vi "Shoot.vi"(5 "Auto_Enable":bool, 6 "Aimed?":bool, 8 "Stopped?":bool, 9 "Yaw":dbl, 11 "Auto_Selection":T1=enum."Ramparts") -> (0 "Far_Shoot":bool, 1 "Hunt":bool, 2 "Shoot":bool, 3 "Auto_Aim":bool, 4 "Lower_Arm":bool, 7 "Auto_Aim_Enable":bool, 10 "Stage":bool)   [LabVIEW 2015]
uses:
  Auto_Selection.ctl
  Shoot_Type_Def.ctl
panel:
  out "error":errorcluster={"status"=TRUE, "code"=0, "source"="DID NOT DRIVE THE DISTANCE : ROUGH TERRAIN"}
  in  "Clear Error":bool
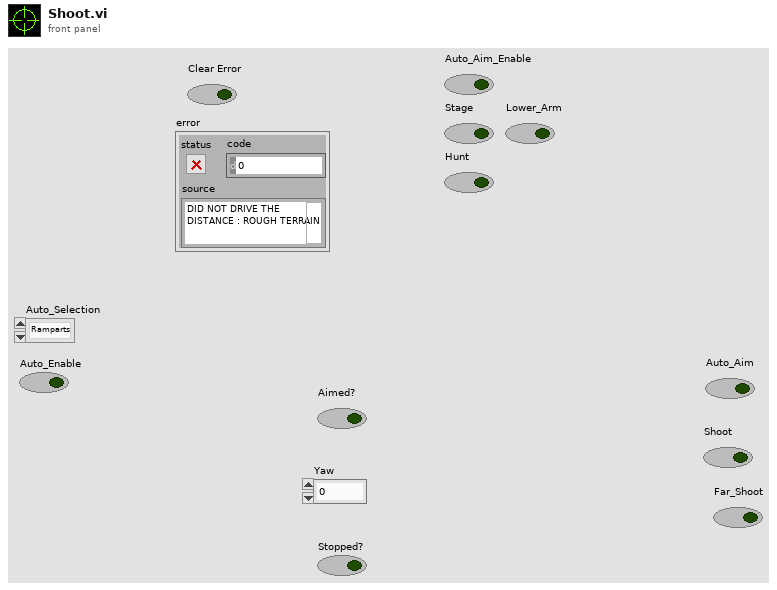
[diagram p1: front panel]
types:
  T1 = typedef "Auto_Selection.ctl" = enum16{"Low Bar", "Rough Terrain", "Rock Wall", "Ramparts", "Moat", "Cheval de Frise", "Portcullis", "None", "One  Ball", "Shoot"}
  T2 = typedef "Shoot_Type_Def.ctl" = enum16{"Off", "Stop", "Shoot", "Aim", "Aim_2", "Delay", "Delay_1"}
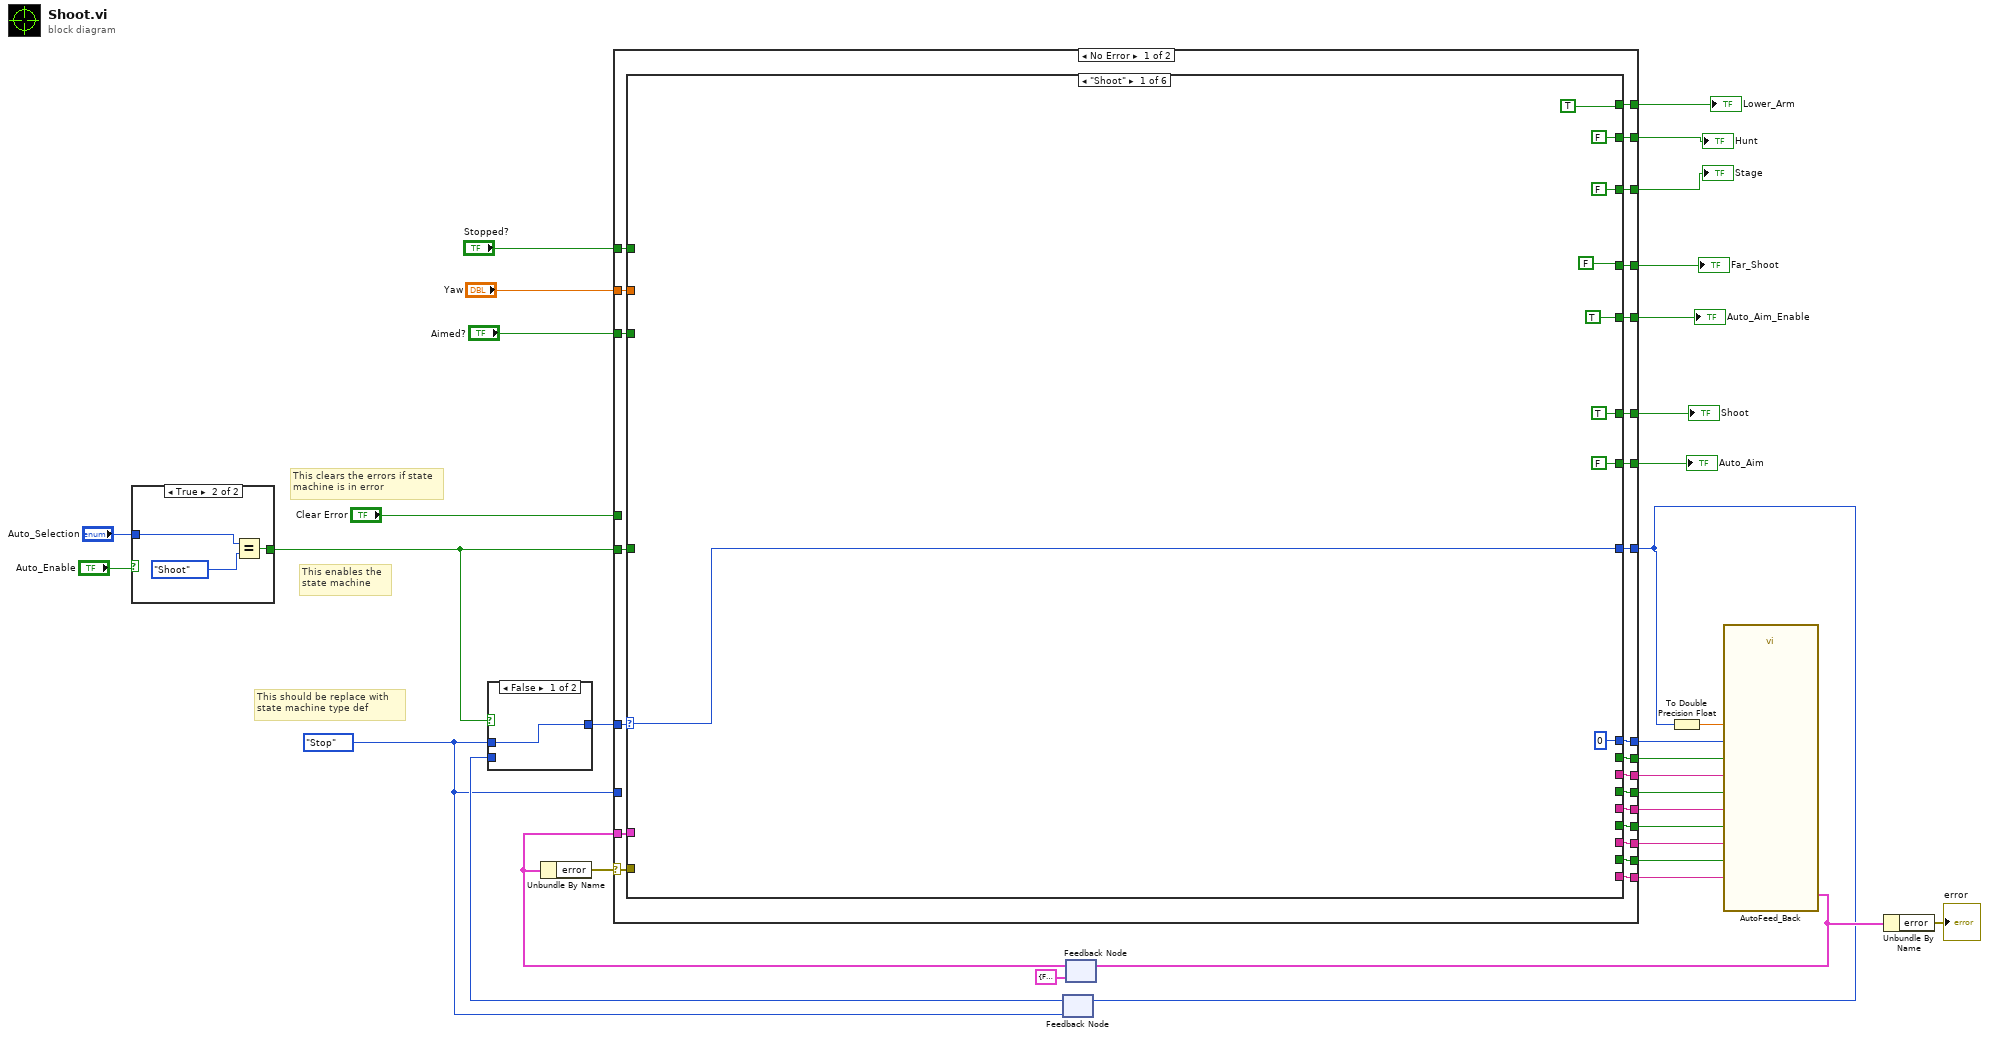
[diagram p0: block diagram]
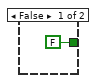
[diagram p2: hidden frame]
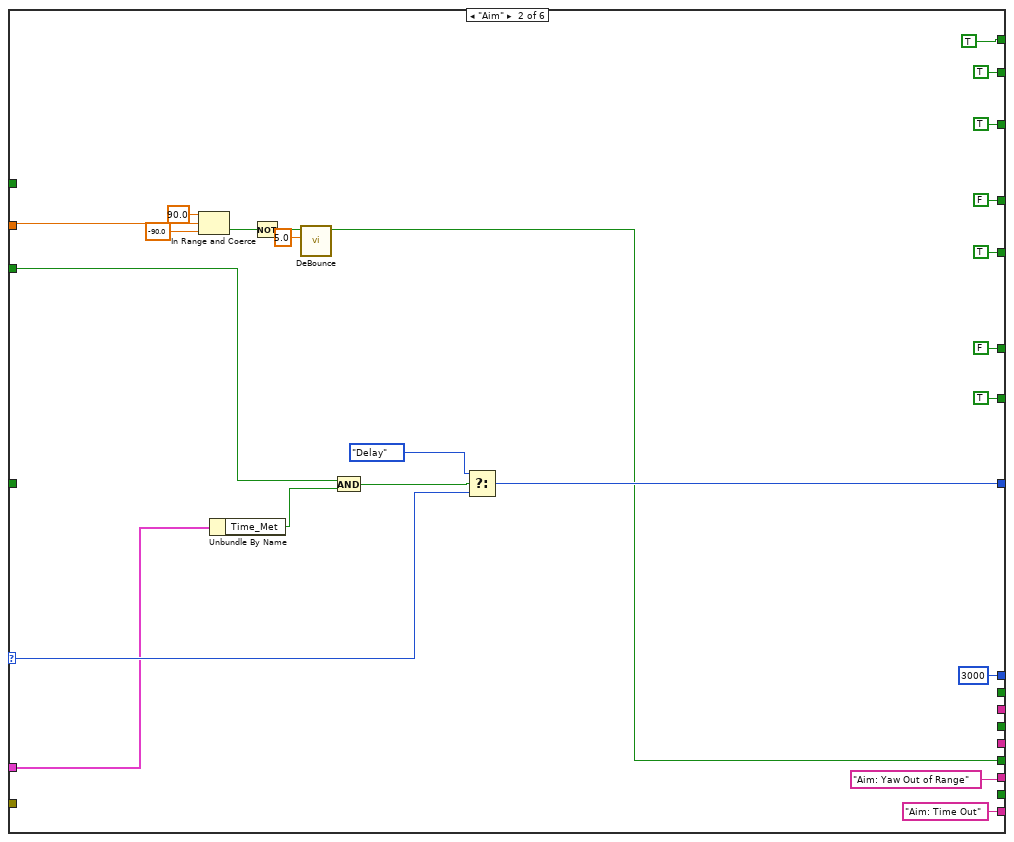
[diagram p4: hidden frame]
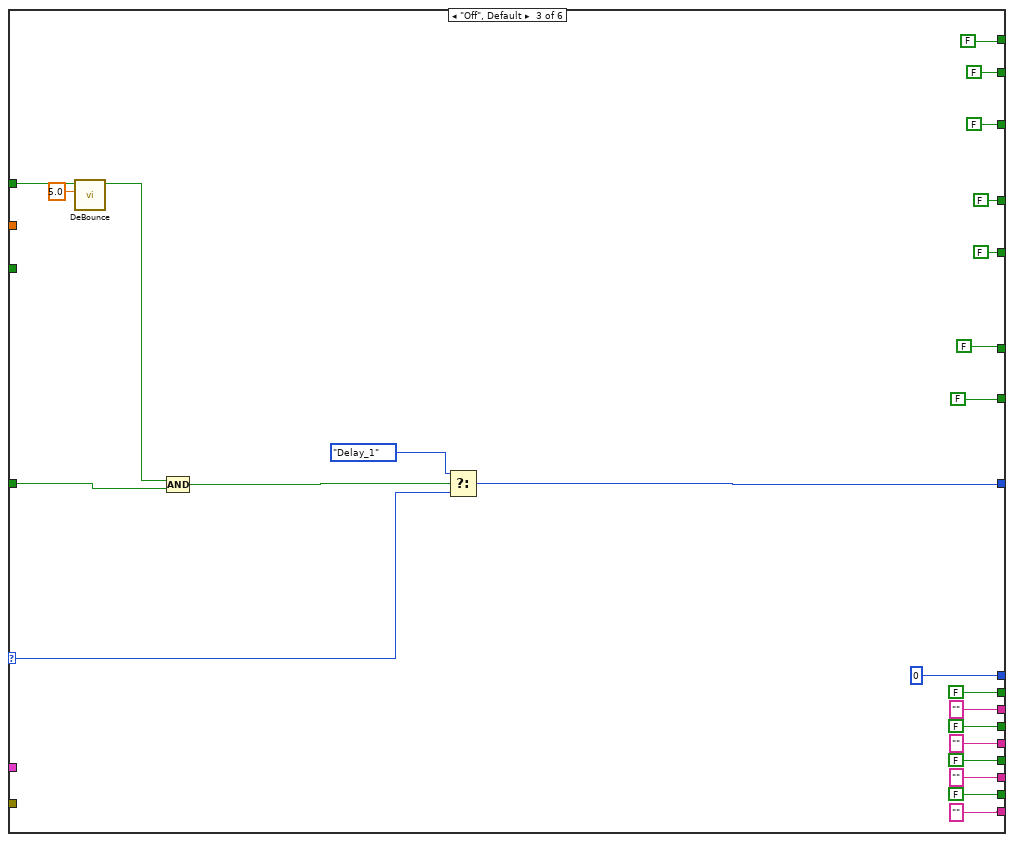
[diagram p5: hidden frame]
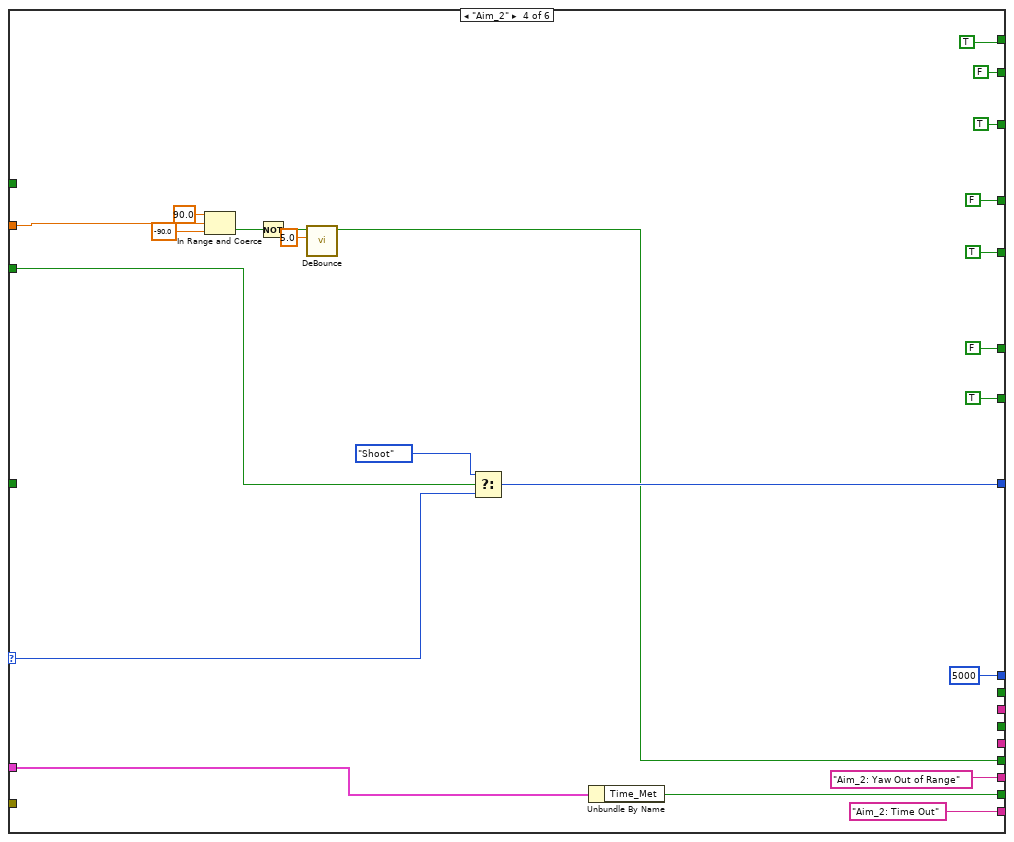
[diagram p6: hidden frame]
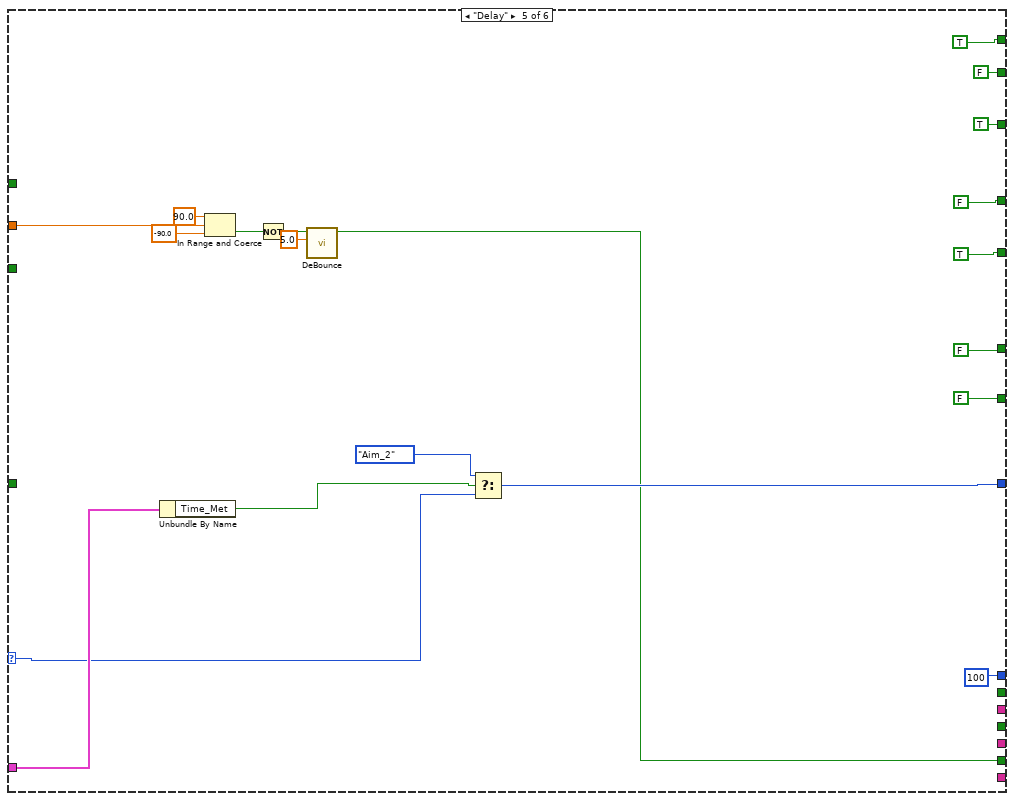
[diagram p7: hidden frame]
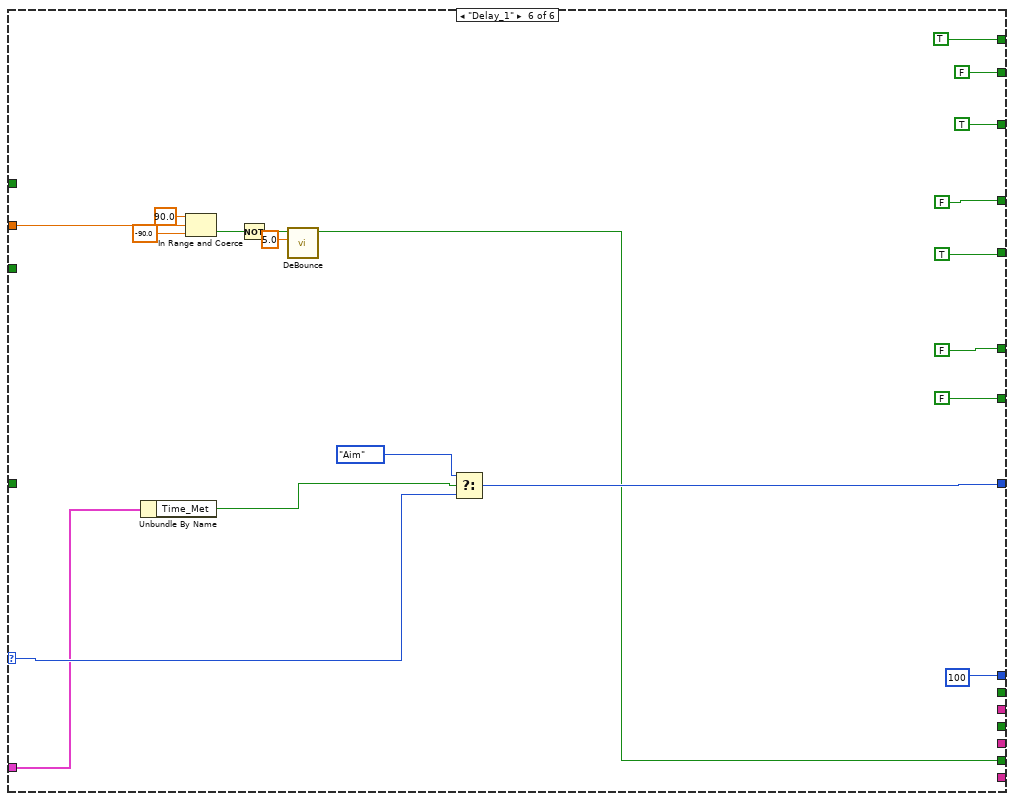
[diagram p8: hidden frame]
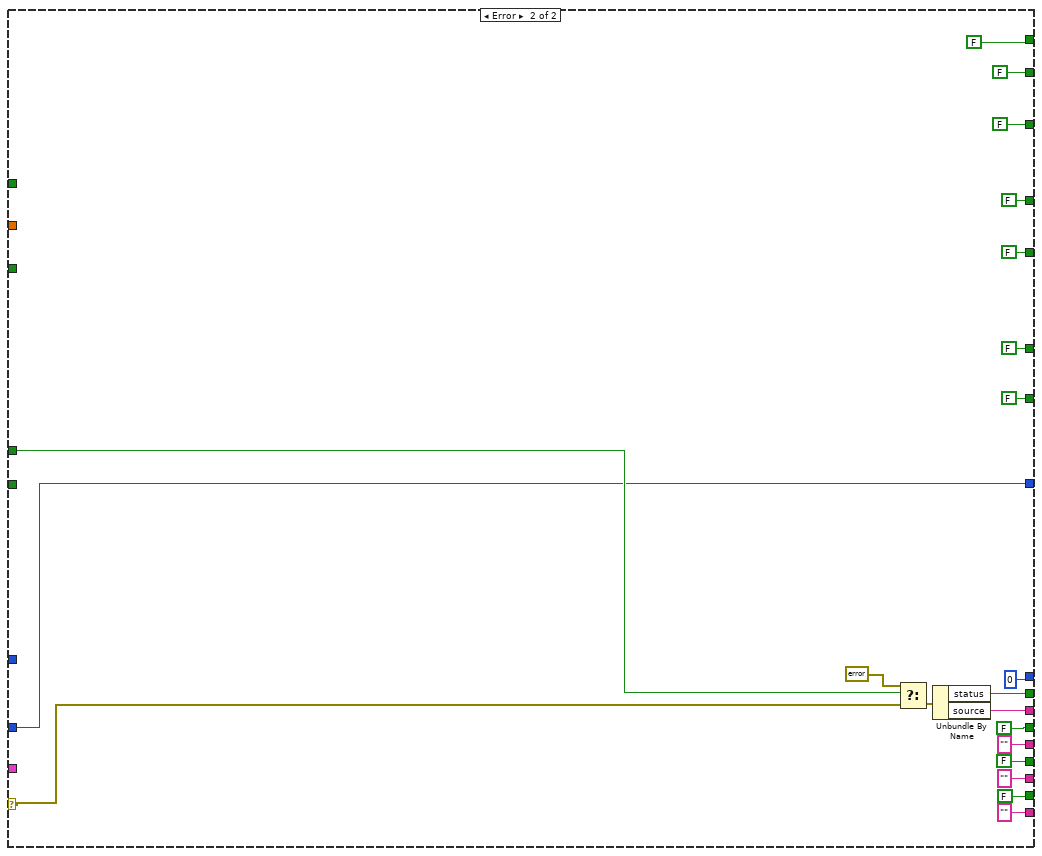
[diagram p9: hidden frame]
diagram:
  w8 = Shoot_Type_Def."Stop"
  # "This clears the errors if state \nmachine is in error"
  # "This enables the \nstate machine"
  # "This should be replace with \nstate machine type def"
  n1 = case shown="True" "Auto_Enable" {
    tunnel: "Auto_Selection" -> [_ w36]
    tunnel: [FALSE w37] -> w25
    frame False {
    }
    frame True {
      n2 = Equal?(x=w36, y=Auto_Selection."Shoot" ("Auto_Selection")) -> (x = y?=w37:bool)
    }
  }
  n3 = feedback #1(w8) -> (w27:T2)
  n4 = case shown="False" w25 {
    tunnel: w8 -> [w38 _]
    tunnel: [w38 w39] -> w28
    tunnel: w27 -> [_ w39]
    frame False {
    }
    frame True {
    }
  }
  n5 = feedback #2(cluster{"Time_Met":bool, "error ":errorcluster} {"Time_Met"=FALSE, "error "={"status"=FALSE, "code"=0, "source"=""}} ("Feedback_State")) -> (w29:cluster{"Time_Met":bool, "error ":errorcluster})
  n6 = Unbundle By Name(w29) -> ("error"=w31:errorcluster)
  n7 = case shown="No Error" w31 {
    selector: w31 -> [w60 w203]
    tunnel: [w63 w200] -> w12
    tunnel: [w62 0] -> w33
    tunnel: "Clear Error" -> [_ w202]
    tunnel: w29 -> [w61 _]
    tunnel: w25 -> [w59 _]
    tunnel: w28 -> [w58 _]
    tunnel: w8 -> [_ w200]
    tunnel: [w57 w198] -> w22
    tunnel: [w56 FALSE] -> w21
    tunnel: [w55 FALSE] -> w20
    tunnel: [w54 FALSE] -> w19
    tunnel: [w53 w197] -> w18
    tunnel: [w52 ""] -> w17
    tunnel: [w51 ""] -> w16
    tunnel: [w50 ""] -> w15
    tunnel: [w49 FALSE] -> w11
    tunnel: [w48 FALSE] -> w10
    tunnel: "Aimed?" -> [w47 _]
    tunnel: "Yaw" -> [w46 _]
    tunnel: [w45 FALSE] -> w6
    tunnel: "Stopped?" -> [w44 _]
    tunnel: [w43 FALSE] -> w4
    tunnel: [w42 FALSE] -> w3
    tunnel: [w41 FALSE] -> w2
    tunnel: [w40 FALSE] -> w1
    frame No Error {
      n8 = case shown="\"Shoot\"" w58 {
        selector: w58 -> [w68 w93 w119 w135 w149 w166]
        tunnel: [0 3000 0 5000 100 100] -> w62
        tunnel: [w68 w92 w118 w133 w153 w169] -> w63
        tunnel: w61 -> [_ w90 _ w134 w150 w165]
        tunnel: w60 -> [_ _ _ _ _ _]
        tunnel: w59 -> [_ _ w105 _ _ _]
        tunnel: [_ _ FALSE _ _ _] -> w57
        tunnel: [_ _ FALSE _ _ _] -> w56
        tunnel: [_ w82 FALSE w126 w152 w168] -> w55
        tunnel: [_ _ FALSE w124 _ _] -> w54
        tunnel: [_ _ "" _ _ _] -> w53
        tunnel: [_ _ "" _ _ _] -> w52
        tunnel: [_ "Aim: Yaw Out of Range" "" "Aim_2: Yaw Out of Range" _ _] -> w51
        tunnel: [_ "Aim: Time Out" "" "Aim_2: Time Out" _ _] -> w50
        tunnel: [FALSE TRUE FALSE TRUE FALSE FALSE] -> w49
        tunnel: [TRUE FALSE FALSE FALSE FALSE FALSE] -> w48
        tunnel: w47 -> [_ w76 _ w136 _ _]
        tunnel: w46 -> [_ w88 _ w137 w148 w164]
        tunnel: [TRUE TRUE FALSE TRUE TRUE TRUE] -> w45
        tunnel: w44 -> [_ _ w103 _ _ _]
        tunnel: [FALSE FALSE FALSE FALSE FALSE FALSE] -> w43
        tunnel: [FALSE TRUE FALSE FALSE FALSE FALSE] -> w42
        tunnel: [FALSE TRUE FALSE TRUE TRUE TRUE] -> w41
        tunnel: [TRUE TRUE FALSE TRUE TRUE TRUE] -> w40
        frame "Shoot" {
        }
        frame "Aim" {
          n9 = In Range and Coerce(upper limit=90.0, x=w88, lower limit=-90.0) -> (In Range?=w85:bool)  [unwired: 1 out]
          n10 = Unbundle By Name(w90) -> ("Time_Met"=w77:bool)
          n11 = Not(x=w85) -> (.not. x?=w84:bool)
          n12 = call "DeBounce.vi"("DB_Count"=5.0, "Value"=w84) -> ("BD_Value"=w82:bool)  [unwired: 9 in]
          n13 = And(x=w76, y=w77) -> (x .and. y?=w78:bool)
          n14 = Select(t=Shoot_Type_Def."Delay", s=w78, f=w93) -> (s? t:f=w92:T2)
        }
        frame "Off", Default {
          n15 = call "DeBounce.vi"("DB_Count"=5.0, "Value"=w103) -> ("BD_Value"=w101:bool)  [unwired: 9 in]
          n16 = Compound Arithmetic op=AND(w101, w105) -> (w104:bool)
          n17 = Select(t=Shoot_Type_Def."Delay_1", s=w104, f=w119) -> (s? t:f=w118:T2)
        }
        frame "Aim_2" {
          n18 = In Range and Coerce(upper limit=90.0, x=w137, lower limit=-90.0) -> (In Range?=w140:bool)  [unwired: 1 out]
          n19 = Not(x=w140) -> (.not. x?=w139:bool)
          n20 = call "DeBounce.vi"("DB_Count"=5.0, "Value"=w139) -> ("BD_Value"=w126:bool)  [unwired: 9 in]
          n21 = Select(t=Shoot_Type_Def."Shoot", s=w136, f=w135) -> (s? t:f=w133:T2)
          n22 = Unbundle By Name(w134) -> ("Time_Met"=w124:bool)
        }
        frame "Delay" {
          n23 = Unbundle By Name(w150) -> ("Time_Met"=w151:bool)
          n24 = In Range and Coerce(upper limit=90.0, x=w148, lower limit=-90.0) -> (In Range?=w160:bool)  [unwired: 1 out]
          n25 = Not(x=w160) -> (.not. x?=w159:bool)
          n26 = call "DeBounce.vi"("DB_Count"=5.0, "Value"=w159) -> ("BD_Value"=w152:bool)  [unwired: 9 in]
          n27 = Select(t=Shoot_Type_Def."Aim_2", s=w151, f=w149) -> (s? t:f=w153:T2)
        }
        frame "Delay_1" {
          n28 = Unbundle By Name(w165) -> ("Time_Met"=w177:bool)
          n29 = In Range and Coerce(upper limit=90.0, x=w164, lower limit=-90.0) -> (In Range?=w180:bool)  [unwired: 1 out]
          n30 = Not(x=w180) -> (.not. x?=w179:bool)
          n31 = call "DeBounce.vi"("DB_Count"=5.0, "Value"=w179) -> ("BD_Value"=w168:bool)  [unwired: 9 in]
          n32 = Select(t=Shoot_Type_Def."Aim", s=w177, f=w166) -> (s? t:f=w169:T2)
        }
      }
    }
    frame Error {
      n33 = Select(t=errorcluster {"status"=FALSE, "code"=0, "source"=""}, s=w202, f=w203) -> (s? t:f=w199:errorcluster)
      n34 = Unbundle By Name(w199) -> ("status"=w198:bool, "source"=w197:string)
    }
  }
  "Auto_Aim" <- w11
  "Shoot" <- w10
  "Auto_Aim_Enable" <- w6
  "Far_Shoot" <- w4
  "Stage" <- w2
  "Hunt" <- w3
  "Lower_Arm" <- w1
  n35 = feedback-in #1(w12) -> ()
  n36 = To Double Precision Float(number=w12) -> (double precision float=w26:dbl)
  n37 = call "AutoFeed_Back.vi"("Code 4"=w15, "Error_4_En"=w19, "Code 3"=w16, "Code 2"=w17, "Error_3_En"=w20, "Error_2_En"=w21, "Code 1"=w18, "Error_1_En"=w22, "Time (ms)"=w33, "State"=w26) -> ("Feedback_State"=w14:cluster{"Time_Met":bool, "error ":errorcluster})  [unwired: 1 in]
  n38 = feedback-in #2(w14) -> ()
  n39 = Unbundle By Name(w14) -> ("error"=→"error":errorcluster)
